vi "Dryer Power Latches.vi"(9 "Time Limit in Seconds":dbl=30.0, 10 "Power On":bool, 11 "Init?":bool) -> (1 "Time of Last Power On":dbl, 2 "Power Off One Shot":bool, 3 "Power On One Shot":bool)   [LabVIEW 2012]
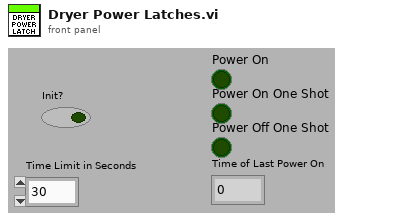
[diagram p1: front panel]
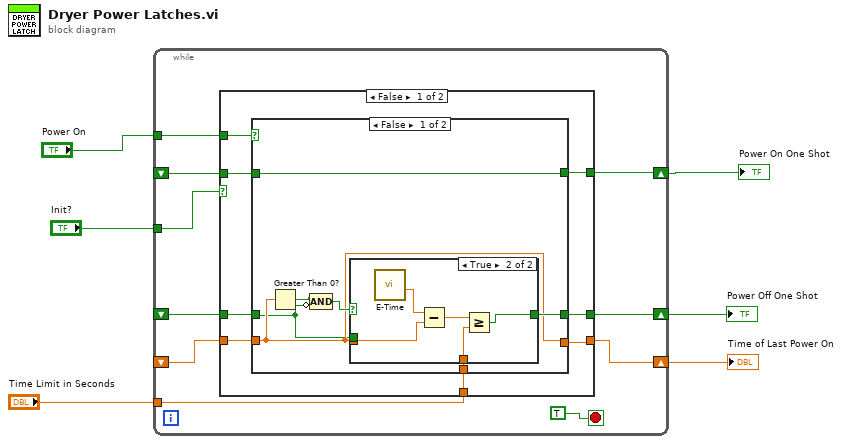
[diagram p0: block diagram]
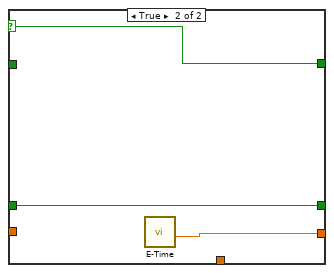
[diagram p3: hidden frame]
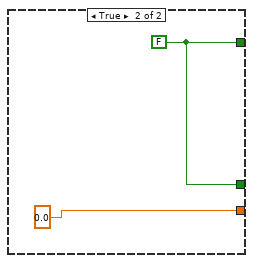
[diagram p4: hidden frame]
diagram:
  n1 = while {
    shift-right: [w15] -> w5
    shift-left: _ -> [w14]
    tunnel: "Power On" -> [w13]
    shift-right: [w12] -> w4
    shift-left: _ -> [w11]
    shift-right: [w10] -> w3
    shift-left: _ -> [w8]
    tunnel: "Time Limit in Seconds" -> [w9]
    tunnel: "Init?" -> [w7]
    stop <- TRUE stop-if-true
    n2 = case shown="False" w7 {
      tunnel: [w23 w42] -> w15
      tunnel: w14 -> [w22 _]
      tunnel: w13 -> [w24 _]
      tunnel: [w21 0.0 ("Elapsed Time (sec)")] -> w12
      tunnel: w11 -> [w18 _]
      tunnel: [w20 w42] -> w10
      tunnel: w8 -> [w19 _]
      tunnel: w9 -> [w17 _]
      frame False {
        n3 = case shown="False" w24 {
          selector: w24 -> [_ w40]
          tunnel: [w31 w40] -> w23
          tunnel: w22 -> [w31 _]
          tunnel: [w27 w39] -> w21
          tunnel: [w29 w38] -> w20
          tunnel: w19 -> [w25 w38]
          tunnel: w18 -> [w27 _]
          tunnel: w17 -> [w30 _]
          frame False {
            n4 = Greater Than 0?(x=w27) -> (x > 0?=w26:bool)
            n5 = Compound Arithmetic op=AND(w26, invert w25) -> (w28:bool)
            n6 = case shown="True" w28 {
              tunnel: w27 -> [_ w36]
              tunnel: w30 -> [_ w34]
              tunnel: [w32 w33] -> w29
              tunnel: w25 -> [w32 _]
              frame False {
              }
              frame True {
                n7 = call "E-Time.vi"() -> ("Elapsed Time (sec)"=w37:dbl)  [unwired: 9 in, 2 out]
                n8 = Subtract(x=w37, y=w36) -> (x-y=w35:dbl)
                n9 = Greater Or Equal?(x=w35, y=w34) -> (x >= y?=w33:bool)
              }
            }
          }
          frame True {
            n10 = call "E-Time.vi"() -> ("Elapsed Time (sec)"=w39:dbl)  [unwired: 9 in, 2 out]
          }
        }
      }
      frame True {
        w42 = FALSE
      }
    }
  }
  "Power On One Shot" <- w5
  "Power Off One Shot" <- w3
  "Time of Last Power On" <- w4
